vi "cut.vi"() -> ()   [LabVIEW 2017]
uses:
  <vilib>/Waveform/WDTOps.llb/WDT Get Waveform Subset DBL.vi
panel:
  out "CursIdx":i32
  out "Active Cursor":u32
  in  "read_in":bool
  in  "stop":bool
  in  "?":enum32{"file io", "cuting", "validity"}(tab)
  in  "path to binary file":path
  in  "file path (use dialog)":path
  in  "Sec":dbl=60.0
  in  "Start Cursor":timestamp
  in  "cut":bool
  out "X középértéke [g]":dbl
  out "X szórása [g]":dbl
  out "Y szórása [g]":dbl
  out "Y középértéke [g]":dbl
  out "Z szórása [g]":dbl
  out "Z középértéke [g]":dbl
  out "A mûszer fejjel lefele lett felhelyezve":bool
  out "A mûszer fordítva lett felhelyezve":bool
  out "Read in":waveform(dbl)[](graph) caption="beolvasott rész"
  out "Levágott rész":waveform(dbl)[](graph)
  out "read in data":waveform(dbl)[](graph) caption="Hosszanti irányú gyorsulás"
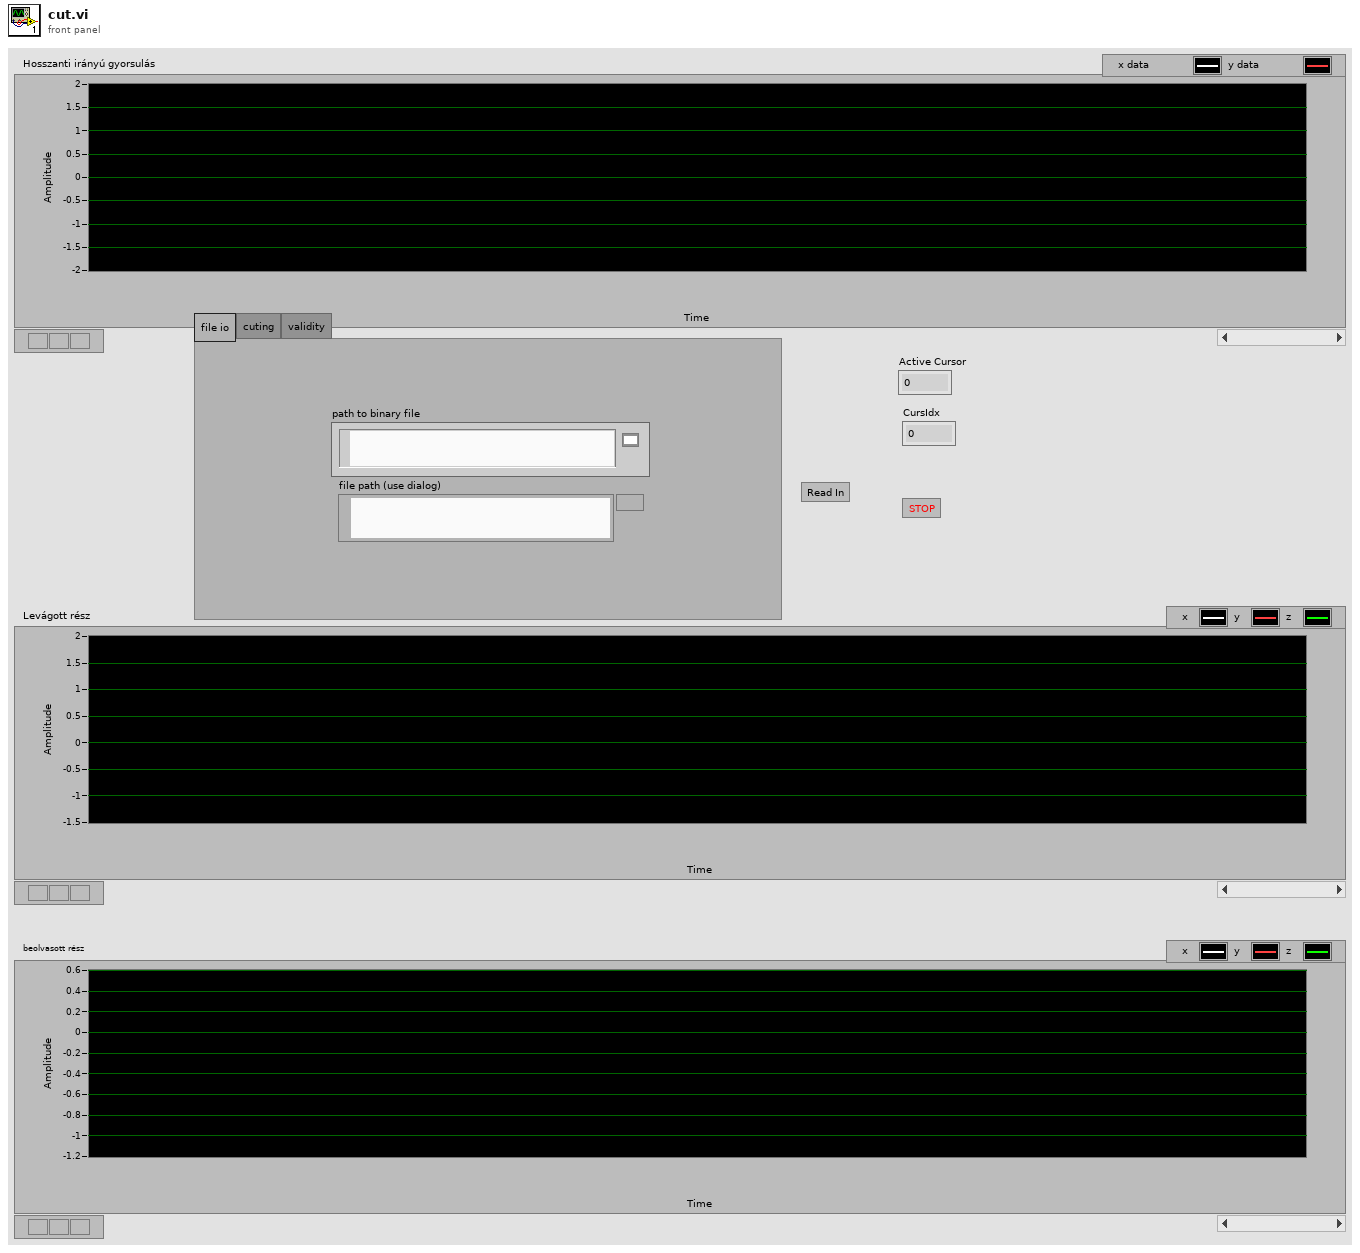
[diagram p1: front panel]
types:
  T1 = typedef "control_time_informations.ctl" = cluster{"starting time":timestamp, "ending time":timestamp, "dt[s]":dbl, "sampling rate [Hz]":dbl, "length":dbl}
  T2 = typedef "control_measurement_settings.ctl" = cluster{"sampling frequency [Hz]":dbl, "measurement interval [± g]":i32, "high precision?":bool, "number of pages":i32, "rate code":i32, "range code":i32, "id":i32}
  T3 = cluster{"statistics":cluster{"mean of x axis acceleration":dbl, "standard devation of x axis acceleration":dbl, "mean of y axis acceleration":dbl, "standard devation of y axis acceleration":dbl, "mean of z axis acceleration":dbl, "standard devation of z axis acceleration":dbl, "mean of magnitude of acceleration":dbl, "standard devation of magnitude of acceleration":dbl}, "time informations":T1, "actigraph settings":T2}
  T4 = enum16{"open", "replace", "create", "open or create", "replace or create", "replace or create with confirmation"}
  T5 = typedef "LVDateTimeRec.ctl" = cluster{"fractional second":dbl, "second":i32, "minute":i32, "hour":i32, "day of month":i32, "month":i32, "year":i32, "day of week":i32, "day of year":i32, "DST":i32}
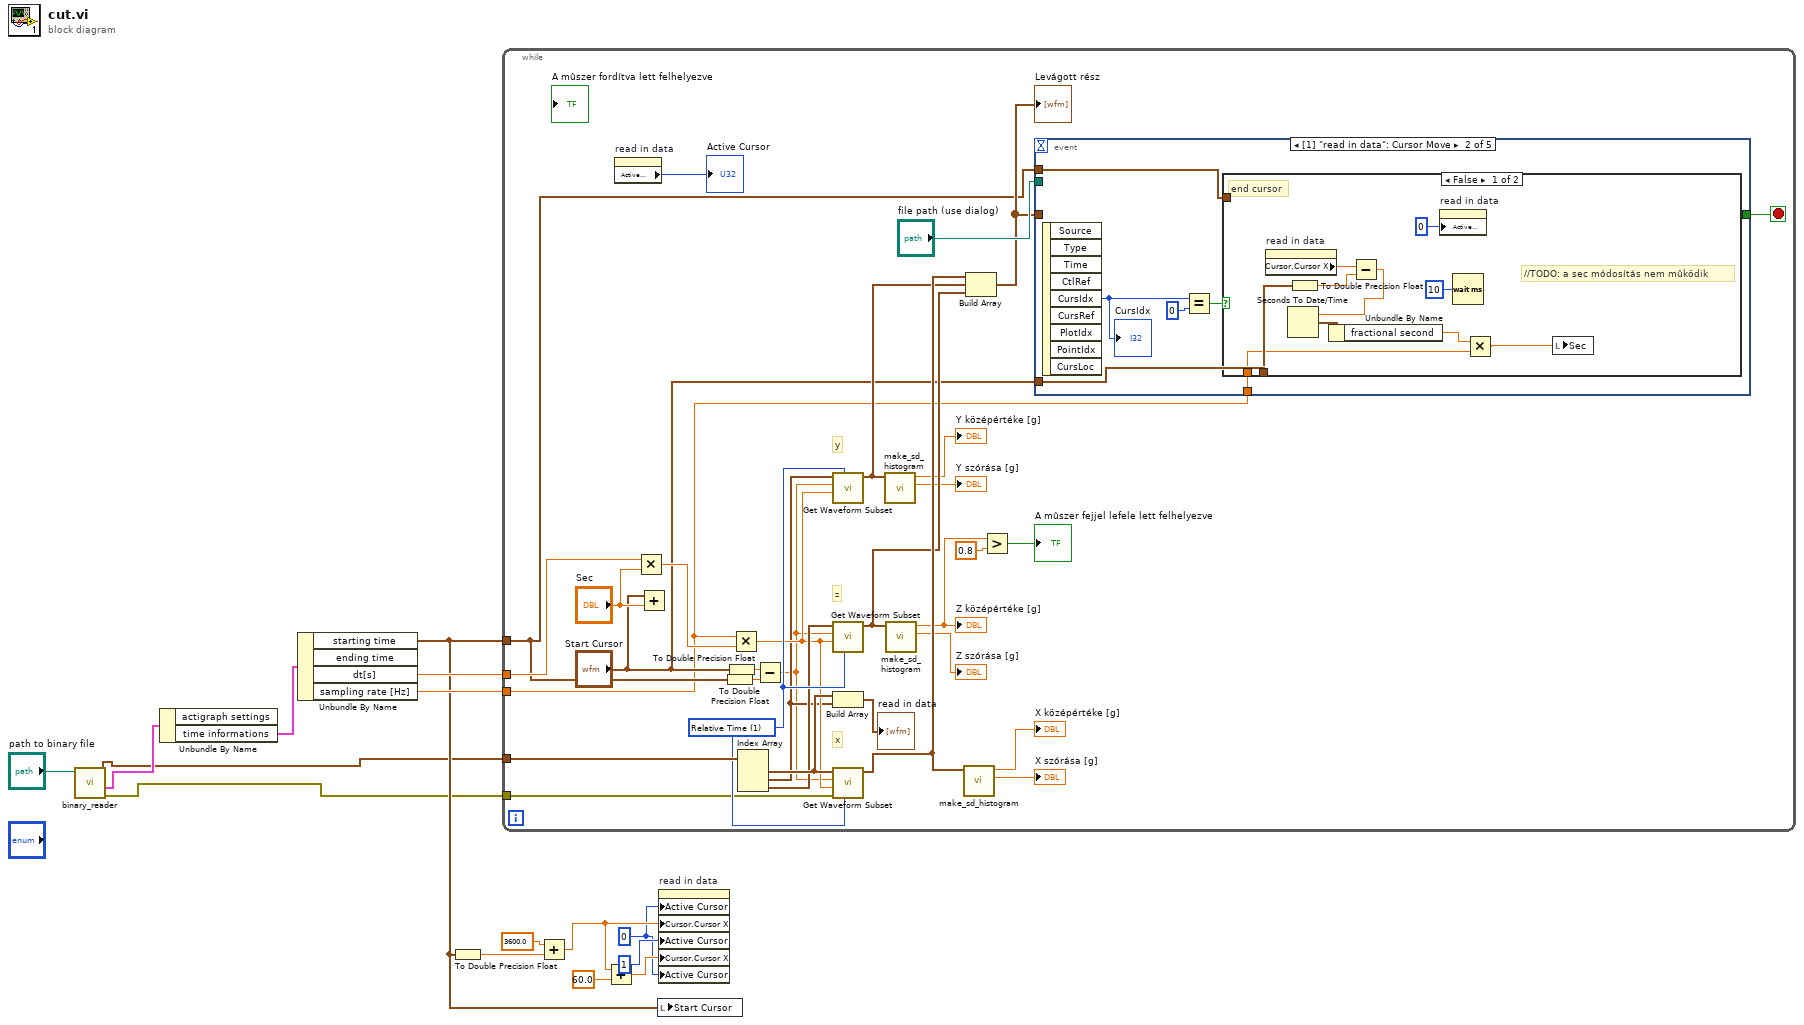
[diagram p0: block diagram]
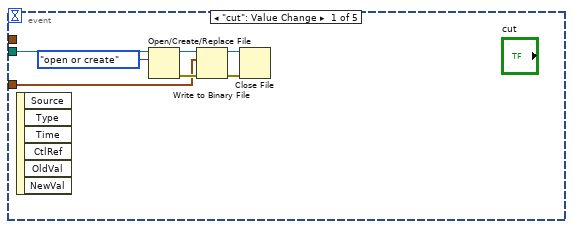
[diagram p2: hidden frame]
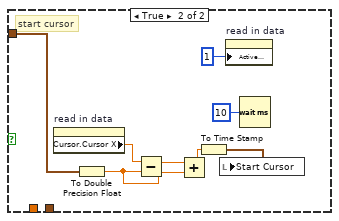
[diagram p3: hidden frame]
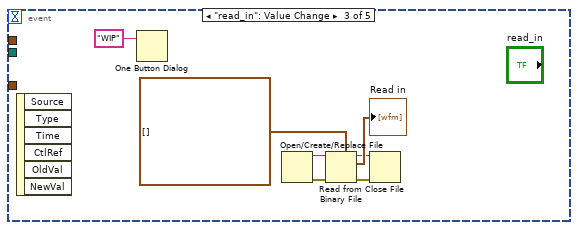
[diagram p4: hidden frame]
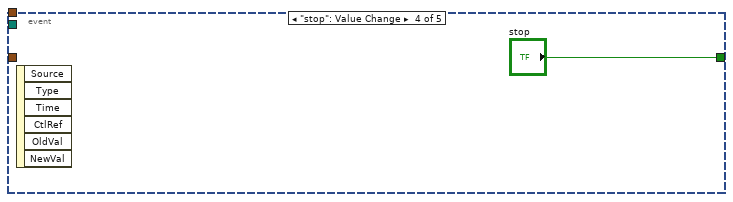
[diagram p5: hidden frame]
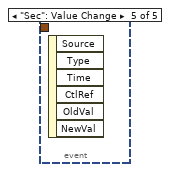
[diagram p6: hidden frame]
diagram:
  w5 = 0
  n1 = call "binary_reader.vi"("path to binary file"="path to binary file") -> ("error out"=w1:errorcluster, "Misc"=w3:T3, "3 axis acceleration in time"=w2:waveform(dbl)[])  [unwired: 6 in, 1 out]
  n2 = Unbundle By Name(w3) -> ("time informations"=w15:T1)  [unwired: 1 out]
  n3 = Unbundle By Name(w15) -> ("starting time"=w9:timestamp, "dt[s]"=w13:dbl, "sampling rate [Hz]"=w14:dbl)  [unwired: 1 out]
  n4 = To Double Precision Float(number=w9) -> (double precision float=w11:dbl)
  n5 = while {
    tunnel: w2 -> [w47]
    tunnel: w1 -> [w31]
    tunnel: w14 -> [w16]
    tunnel: w13 -> [w27]
    tunnel: w9 -> [w18]
    stop <- w24 stop-if-true
    w42 = u16 1 items=["Samples", "Relative Time"] ("start/duration format")
    # "z"
    # "y"
    # "x"
    n6 = property on="read in data" class="WFGraph (strict)"() -> ("Active Cursor"=→"Active Cursor":u32)  [unwired: 2 in, 2 out]
    n7 = Multiply(x=w27, y="Sec") -> (x*y=w29:dbl)
    n8 = Add(x="Start Cursor", y="Sec") -> ()  [unwired: 1 out]
    n9 = To Double Precision Float(number=w18) -> (double precision float=w19:dbl)
    n10 = To Double Precision Float(number="Start Cursor") -> (double precision float=w20:dbl)
    n11 = Multiply(x=w16, y=w29) -> (x*y=w30:dbl)
    n12 = Index Array(array=w47) -> (element #1=w43:waveform(dbl), element #2=w28:waveform(dbl), element #3=w41:waveform(dbl))  [unwired: 3 in]
    n13 = Subtract(x=w20, y=w19) -> (x-y=w17:dbl)
    n14 = call-poly <vilib>:"Get Waveform Subset.vi"("start/duration format"=w42, "duration"=w30, "start samples/time"=w17, "waveform in"=w28) -> ("waveform out"=w39:waveform(dbl))  [unwired: 2 in, 3 out]
    n15 = call-poly <vilib>:"Get Waveform Subset.vi"("start/duration format"=w42, "duration"=w30, "start samples/time"=w17, "waveform in"=w41) -> ("waveform out"=w38:waveform(dbl))  [unwired: 2 in, 3 out]
    n16 = Build Array(w43, w28) -> (→"read in data":waveform(dbl)[])
    n17 = call-poly <vilib>:"Get Waveform Subset.vi"("start/duration format"=w42, "error in (no error)"=w31, "duration"=w30, "start samples/time"=w17, "waveform in"=w43) -> ("waveform out"=w40:waveform(dbl))  [unwired: 1 in, 3 out]
    n18 = call "make_sd_histogram.vi"("waveform"=w39) -> ("Szórás [g]"=→"Y szórása [g]":dbl, "Középérték [g]"=→"Y középértéke [g]":dbl)  [unwired: 4 in, 5 out]
    n19 = call "make_sd_histogram.vi"("waveform"=w38) -> ("Szórás [g]"=→"Z szórása [g]":dbl, "Középérték [g]"=w33:dbl)  [unwired: 4 in, 5 out]
    "Z középértéke [g]" <- w33
    n20 = call "make_sd_histogram.vi"("waveform"=w40) -> ("Szórás [g]"=→"X szórása [g]":dbl, "Középérték [g]"=→"X középértéke [g]":dbl)  [unwired: 4 in, 5 out]
    n21 = Build Array(w40, w39, w38) -> (w25:waveform(dbl)[])
    "Levágott rész" <- w25
    n22 = Greater?(x=w33, y=0.8) -> (0:→"A mûszer fejjel lefele lett felhelyezve":bool)
    n23 = event shown="[1] \"read in data\": Cursor Move" {
      selector: _ -> [_ _ _ _ _]
      dyn-events: _ -> [_ _ _ _ _]
      timeout: _ -> [_ _ _ _ _]
      tunnel: [_ _ _ "stop" _] -> w24
      tunnel: "file path (use dialog)" -> [w50 _ _ _ _]
      tunnel: w25 -> [w49 _ _ _ _]
      tunnel: w18 -> [_ w57 _ _ _]
      tunnel: "Start Cursor" -> [_ w56 _ _ _]
      tunnel: w16 -> [_ w55 _ _ _]
      event "cut": Value Change {
        n24 = event-data() -> ()  [unwired: 1 in, 6 out]
        n25 = Open/Create/Replace File(file path (use dialog)=w50, operation (0:open)=T4."open or create") -> (refnum out=w52:refnum<file>, error out=w51:errorcluster)  [unwired: 4 in, 1 out]
        n26 = Write to Binary File(file (use dialog)=w52, data=w49, error in=w51) -> (refnum out=w54:refnum<file>, error out=w53:errorcluster)  [unwired: 3 in, 1 out]
        n27 = Close File(refnum=w54, error in=w53) -> ()  [unwired: 2 out]
      }
      event "read in data": Cursor Move {
        n28 = event-data() -> ("CursIdx"=w60:i32)  [unwired: 1 in, 8 out]
        "CursIdx" <- w60
        n29 = Equal?(x=w60, y=0) -> (x = y?=w58:bool)
        n30 = case shown="False" w58 {
          tunnel: w57 -> [_ w75]
          tunnel: w56 -> [w67 _]
          tunnel: w55 -> [w63 _]
          frame False {
            # "//TODO: a sec módosítás nem mûködik"
            # "end cursor"
            n31 = property on="read in data" class="WFGraph (strict)"() -> ("Cursor.Cursor X"=w69:dbl)  [unwired: 2 in, 2 out]
            n32 = To Double Precision Float(number=w67) -> (double precision float=w68:dbl)
            n33 = Subtract(x=w69, y=w68) -> (x-y=w65:dbl)
            n34 = Seconds To Date/Time(time stamp (now)=w65) -> (date time rec=w64:T5)  [unwired: 1 in]
            n35 = Unbundle By Name(w64) -> ("fractional second"=w62:dbl)
            n36 = property on="read in data" class="WFGraph (strict)"("Active Cursor"=0) -> ()  [unwired: 2 in, 2 out]
            n37 = Wait (ms)(milliseconds to wait=u32 10) -> ()  [unwired: 1 out]
            n38 = Multiply(x=w62, y=w63) -> (x*y=w61:dbl)
            n39 = local write "Sec"(w61) -> ()
          }
          frame True {
            # "start cursor"
            n40 = property on="read in data" class="WFGraph (strict)"() -> ("Cursor.Cursor X"=w78:dbl)  [unwired: 2 in, 2 out]
            n41 = To Double Precision Float(number=w75) -> (double precision float=w73:dbl)
            n42 = Subtract(x=w78, y=w73) -> (x-y=w74:dbl)
            n43 = Add(x=w74, y=w73) -> (x+y=w71:dbl)
            n44 = To Time Stamp(1:w71) -> (0:w72:timestamp)
            n45 = local write "Start Cursor"(w72) -> ()
            n46 = property on="read in data" class="WFGraph (strict)"("Active Cursor"=1) -> ()  [unwired: 2 in, 2 out]
            n47 = Wait (ms)(milliseconds to wait=u32 10) -> ()  [unwired: 1 out]
          }
        }
      }
      event "read_in": Value Change {
        n48 = event-data() -> ()  [unwired: 1 in, 6 out]
        n49 = One Button Dialog(message="WIP") -> ()  [unwired: 1 in, 1 out]
        n50 = Open/Create/Replace File() -> (refnum out=w83:refnum<file>, error out=w81:errorcluster)  [unwired: 6 in, 1 out]
        n51 = Read from Binary File(5:waveform(dbl)[] [] ("appended array"), 8:w81, 11:w83) -> (0:w82:errorcluster, 2:→"Read in":waveform(dbl)[], 3:w80:refnum<file>)  [unwired: 3 in, 1 out]
        n52 = Close File(refnum=w80, error in=w82) -> ()  [unwired: 2 out]
      }
      event "stop": Value Change {
        n53 = event-data() -> ()  [unwired: 1 in, 6 out]
      }
      event "Sec": Value Change {
        n54 = event-data() -> ()  [unwired: 1 in, 6 out]
      }
    }
  }
  n55 = Add(x=3600.0, y=w11) -> (x+y=w8:dbl)
  n56 = Add(x=w8, y=60.0) -> (x+y=w6:dbl)
  n57 = local write "Start Cursor"(w9) -> ()
  n58 = property on="read in data" class="WFGraph (strict)"("Active Cursor"=w5, "Cursor.Cursor X"=w8, "Active Cursor"=1, "Cursor.Cursor X"=w6, "Active Cursor"=w5) -> ()  [unwired: 2 in, 2 out]
